vi "Strip Unit.vi"(8 "错误输入":errorcluster, 10 "Number or 1D array with units":variant) -> (0 "错误输出":errorcluster, 2 "Pure Number(s) (base units)":variant)   [LabVIEW 2012, in "TD Tools.lvlib"]
uses:
  TD Tools.lvlib
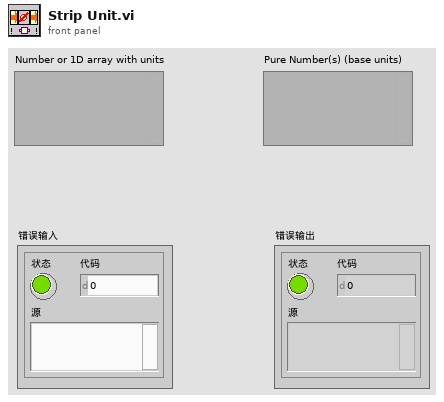
[diagram p1: front panel]
types:
  T1 = typedef "TD Tools.lvlib/Type Descriptor.ctl" = u16[]
  T2 = typedef "TD Tools.lvlib/Type Descriptor Header.ctl" = cluster{"length":u16, "private":u8, "type":T3, "# elements":u16}
  T3 = typedef "TD Tools.lvlib/Type Descriptor Enumeration.ctl" = enum16{"<Null>", "I8", "I16", "I32", "I64", "U8", "U16", "U32", "U64", "SGL", "DBL", "EXT", "CSG", "CDB", "CXT", "0x0F", "0x10", "0x11", "0x12", "0x13", "0x14", "Enum U8", "Enum U16", "Enum U32", "Enum U64", "SGL PQ", "DBL PQ", "EXT PQ", "CSG PQ", "CDB PQ", "CXT PQ", "0x1F", "0x20", "Boolean", "0x22", "0x23", "0x24", "0x25", "0x26", "0x27", "0x28", "0x29", "0x2A", "0x2B", "0x2C", "0x2D", "0x2E", "0x2F", "String", "0x31", "Path", "Pict", "0x34", "0x35", "0x36", "DAQ", "0x38", "0x39", "0x3A", "0x3B", "0x3C", "0x3D", "0x3E", "0x3F", "Array", "0x41", "0x42", "0x43", "0x44", "0x45", "0x46", "0x47", "0x48", "0x49", "0x4A", "0x4B", "0x4C", "0x4D", "0x4E", "0x4F", "Cluster", "0x51", "0x52", "Variant", "Waveform", "0x55", "0x56", "0x57", "0x58", "0x59", "0x5A", "0x5B", "0x5C", "0x5D", "0x5E", "0x5F", "0x60", "0x61", "0x62", "0x63", "0x64", "0x65", "0x66", "0x67", "0x68", "0x69", "0x6A", "0x6B", "0x6C", "0x6D", "0x6E", "0x6F", "Refnum"}
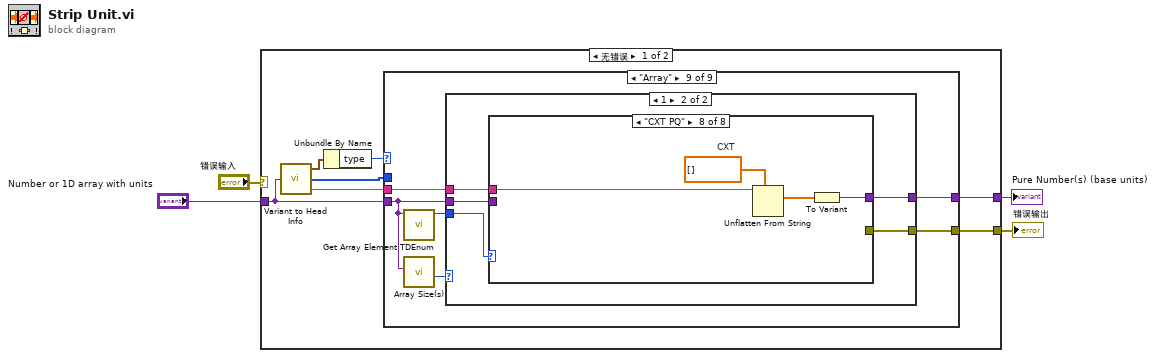
[diagram p0: block diagram]
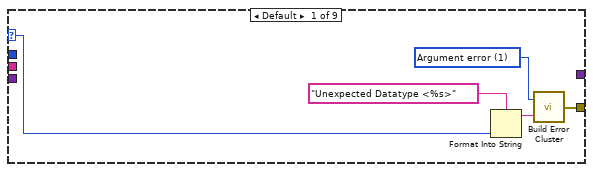
[diagram p2: hidden frame]
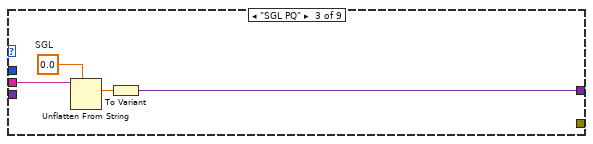
[diagram p4: hidden frame]
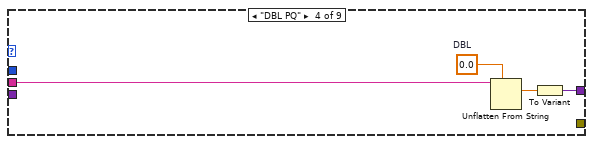
[diagram p5: hidden frame]
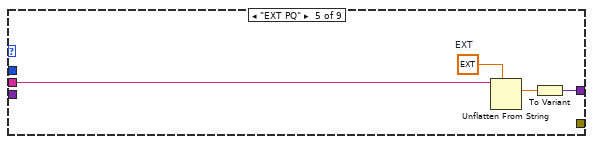
[diagram p6: hidden frame]
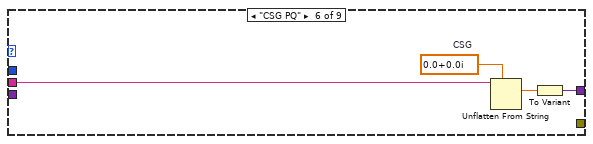
[diagram p7: hidden frame]
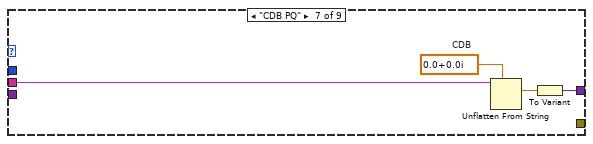
[diagram p8: hidden frame]
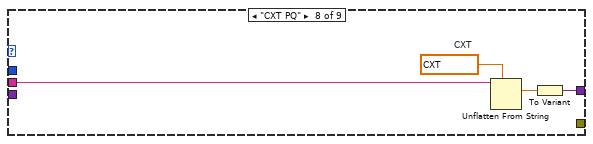
[diagram p9: hidden frame]
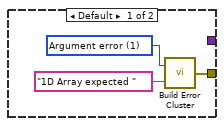
[diagram p10: hidden frame]
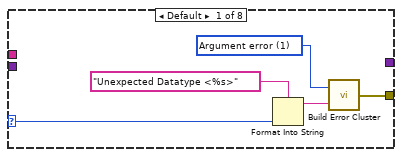
[diagram p11: hidden frame]
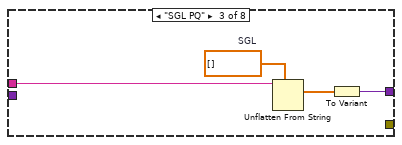
[diagram p13: hidden frame]
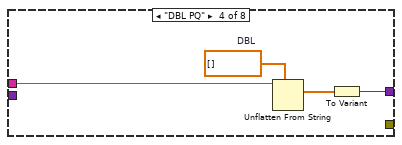
[diagram p14: hidden frame]
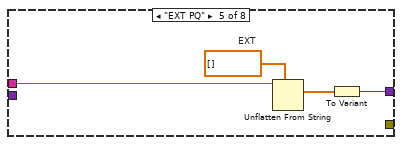
[diagram p15: hidden frame]
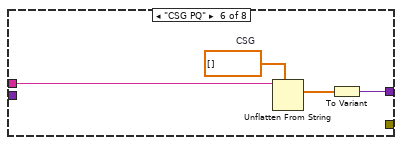
[diagram p16: hidden frame]
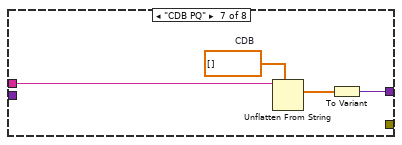
[diagram p17: hidden frame]
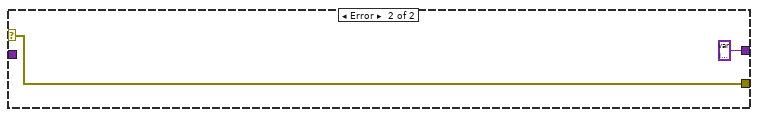
[diagram p18: hidden frame]
diagram:
  n1 = case shown="无错误" "错误输入" {
    selector: "错误输入" -> [_ w87]
    tunnel: [w11 w87] -> w2
    tunnel: "Number or 1D array with units" -> [w5 _]
    tunnel: [w6 variant ("Variant")] -> w3
    frame No Error {
      n2 = call "Variant to Head Info.vi"("Variant"=w5) -> ("Data String"=w7:string, "Type Descriptor"=w8:T1, "Type Descriptor Header"=w10:T2)  [unwired: 2 in]
      n3 = Unbundle By Name(w10) -> ("type"=w9:T3)
      n4 = case shown="\"Array\"" w9 {
        selector: w9 -> [w13 _ _ _ _ _ _ _ _]
        tunnel: [w16 _ _ _ _ _ _ _ w46] -> w11
        tunnel: w8 -> [_ _ _ _ _ _ _ _ _]
        tunnel: w7 -> [_ _ w18 w22 w26 w30 w34 w38 w44]
        tunnel: [_ w17 w19 w23 w27 w31 w35 w39 w45] -> w6
        tunnel: w5 -> [_ w17 _ _ _ _ _ _ w43]
        frame Default {
          w15 = 1 items=["No error", "Argument error", "Memory is full", "Out of zone", "End of file", "File already open", "Generic file I/O error", "File not found", "File permission error", "Disk is full", "Duplicate path", "Too many files open", "System feature not enabled", "Resource file not found", "Cannot add resource", "Resource not found", "Image not found", "Image memory error", "Pen does not exist", "Config type invalid", "Config token not found", "Config parse error", "Config memory error", "Bad external code format", "Bad external code offset", "External code not present", "Null window", "Destroy window error", "Null menu", "Print aborted", "Bad print record", "Print driver error", "Windows error during printing", "Memory error during printing", "Print dialog error", "Generic print error", "Invalid device refnum", "Device not found", "Device parameter error", "Device unit error", "Cannot open device", "Device call aborted", "Generic error", "Cancelled by user", "Object ID too low", "Object ID too high", "Object not in heap", "Unknown heap", "Unknown object (invalid DefProc)", "Unknown object (DefProc not in table)", "Message out of range", "Invalid (null) method", "Unknown message", "Manager call not supported", "Bad address", "Network operation in progress", "Network operation timed out", "Connection is busy", "Network attribute not supported", "Network error", "Address in use", "System out of memory", "Connection aborted", "Connection refused", "Not connected", "Already connected", "Connection closed", "Initialization error (interapplication manager)", "Bad occurrence", "Wait on unbound occurrence handler", "Occurrence queue overflow", "Datalog type conflict", "Unused", "Unrecognized type (interapplication manager)", "Memory corrupt", "Failed to make temporary DLL", "Old CIN version", "Drag socket not found", "Failed to load drop-object", "Failed to register OLE object", "Failed to release OLE object", "Format specifier type mismatch", "Unknown format specifier", "Too few format specifiers", "Too many format specifiers", "Scan failed", "Newer CIN version", "Error converting to variant", "Runtime menu error", "Password tampered", "Variant attribute not found", "Incompatible variant data type", "Event data is not available", "Event Store is not present", "Occurrence is not found", "Event Queue is not created", "Event info is not available", "Refnum passed is NULL", "Error retrieving Class GUID", "Error retrieving CoClass GUID", "Error retrieving TypeLib GUID.", "Bad built application magic bytes.", "Specific driver is different from the specific driver associated with the Logical Name.", "There is no session opened to the class driver.", "Max Error", "MAX - Error with config objects", "MAX - Error loading configuration", "MAX - Group not supported"]
          n5 = Format Into String(format string="Unexpected Datatype <%s>" ("Format String"), w13) -> (resulting string=w12:string)  [unwired: 2 in, 1 out]
          n6 = call "Build Error Cluster.vi"("String to Prepend to source (\"\")"=w12, "code"=w15) -> ("error out"=w16:errorcluster)
        }
        frame "SGL".."CXT" {
        }
        frame "SGL PQ" {
          w21 = sgl 0.0  # SGL
          n7 = Unflatten From String(type=w21, binary string=w18) -> (value=w20:sgl)  [unwired: 3 in, 2 out]
          n8 = To Variant(anything=w20) -> (Variant=w19:variant)
        }
        frame "DBL PQ" {
          w25 = 0.0  # DBL
          n9 = Unflatten From String(type=w25, binary string=w22) -> (value=w24:dbl)  [unwired: 3 in, 2 out]
          n10 = To Variant(anything=w24) -> (Variant=w23:variant)
        }
        frame "EXT PQ" {
          w29 = ext 0.0  # EXT
          n11 = Unflatten From String(type=w29, binary string=w26) -> (value=w28:ext)  [unwired: 3 in, 2 out]
          n12 = To Variant(anything=w28) -> (Variant=w27:variant)
        }
        frame "CSG PQ" {
          w33 = csg 0.0+0.0i  # CSG
          n13 = Unflatten From String(type=w33, binary string=w30) -> (value=w32:csg)  [unwired: 3 in, 2 out]
          n14 = To Variant(anything=w32) -> (Variant=w31:variant)
        }
        frame "CDB PQ" {
          w37 = cdb 0.0+0.0i  # CDB
          n15 = Unflatten From String(type=w37, binary string=w34) -> (value=w36:cdb)  [unwired: 3 in, 2 out]
          n16 = To Variant(anything=w36) -> (Variant=w35:variant)
        }
        frame "CXT PQ" {
          w41 = cxt 0.0+0.0i  # CXT
          n17 = Unflatten From String(type=w41, binary string=w38) -> (value=w40:cxt)  [unwired: 3 in, 2 out]
          n18 = To Variant(anything=w40) -> (Variant=w39:variant)
        }
        frame "Array" {
          n19 = call "Get Array Element TDEnum.vi"("Array"=w43) -> ("Type Code"=w47:T3)  [unwired: 9 in, 1 out]
          n20 = call "Array Size(s).vi"("Array"=w43) -> ("N dims"=w42:u32)  [unwired: 8 in, 2 out]
          n21 = case shown="1" w42 {
            tunnel: w47 -> [_ w55]
            tunnel: [w49 w54] -> w46
            tunnel: [_ w53] -> w45
            tunnel: w44 -> [_ w52]
            tunnel: w43 -> [_ w51]
            frame Default {
              w50 = 1 items=["No error", "Argument error", "Memory is full", "Out of zone", "End of file", "File already open", "Generic file I/O error", "File not found", "File permission error", "Disk is full", "Duplicate path", "Too many files open", "System feature not enabled", "Resource file not found", "Cannot add resource", "Resource not found", "Image not found", "Image memory error", "Pen does not exist", "Config type invalid", "Config token not found", "Config parse error", "Config memory error", "Bad external code format", "Bad external code offset", "External code not present", "Null window", "Destroy window error", "Null menu", "Print aborted", "Bad print record", "Print driver error", "Windows error during printing", "Memory error during printing", "Print dialog error", "Generic print error", "Invalid device refnum", "Device not found", "Device parameter error", "Device unit error", "Cannot open device", "Device call aborted", "Generic error", "Cancelled by user", "Object ID too low", "Object ID too high", "Object not in heap", "Unknown heap", "Unknown object (invalid DefProc)", "Unknown object (DefProc not in table)", "Message out of range", "Invalid (null) method", "Unknown message", "Manager call not supported", "Bad address", "Network operation in progress", "Network operation timed out", "Connection is busy", "Network attribute not supported", "Network error", "Address in use", "System out of memory", "Connection aborted", "Connection refused", "Not connected", "Already connected", "Connection closed", "Initialization error (interapplication manager)", "Bad occurrence", "Wait on unbound occurrence handler", "Occurrence queue overflow", "Datalog type conflict", "Unused", "Unrecognized type (interapplication manager)", "Memory corrupt", "Failed to make temporary DLL", "Old CIN version", "Drag socket not found", "Failed to load drop-object", "Failed to register OLE object", "Failed to release OLE object", "Format specifier type mismatch", "Unknown format specifier", "Too few format specifiers", "Too many format specifiers", "Scan failed", "Newer CIN version", "Error converting to variant", "Runtime menu error", "Password tampered", "Variant attribute not found", "Incompatible variant data type", "Event data is not available", "Event Store is not present", "Occurrence is not found", "Event Queue is not created", "Event info is not available", "Refnum passed is NULL", "Error retrieving Class GUID", "Error retrieving CoClass GUID", "Error retrieving TypeLib GUID.", "Bad built application magic bytes.", "Specific driver is different from the specific driver associated with the Logical Name.", "There is no session opened to the class driver.", "Max Error", "MAX - Error with config objects", "MAX - Error loading configuration", "MAX - Group not supported"]
              n22 = call "Build Error Cluster.vi"("String to Prepend to source (\"\")"="1D Array expected " ("Format String"), "code"=w50) -> ("error out"=w49:errorcluster)
            }
            frame 1 {
              n23 = case shown="\"CXT PQ\"" w55 {
                selector: w55 -> [w57 _ _ _ _ _ _ _]
                tunnel: [w56 _ _ _ _ _ _ _] -> w54
                tunnel: [_ w61 w62 w66 w70 w74 w78 w82] -> w53
                tunnel: w51 -> [_ w61 _ _ _ _ _ _]
                tunnel: w52 -> [_ _ w63 w67 w71 w75 w79 w83]
                frame Default {
                  w60 = 1 items=["No error", "Argument error", "Memory is full", "Out of zone", "End of file", "File already open", "Generic file I/O error", "File not found", "File permission error", "Disk is full", "Duplicate path", "Too many files open", "System feature not enabled", "Resource file not found", "Cannot add resource", "Resource not found", "Image not found", "Image memory error", "Pen does not exist", "Config type invalid", "Config token not found", "Config parse error", "Config memory error", "Bad external code format", "Bad external code offset", "External code not present", "Null window", "Destroy window error", "Null menu", "Print aborted", "Bad print record", "Print driver error", "Windows error during printing", "Memory error during printing", "Print dialog error", "Generic print error", "Invalid device refnum", "Device not found", "Device parameter error", "Device unit error", "Cannot open device", "Device call aborted", "Generic error", "Cancelled by user", "Object ID too low", "Object ID too high", "Object not in heap", "Unknown heap", "Unknown object (invalid DefProc)", "Unknown object (DefProc not in table)", "Message out of range", "Invalid (null) method", "Unknown message", "Manager call not supported", "Bad address", "Network operation in progress", "Network operation timed out", "Connection is busy", "Network attribute not supported", "Network error", "Address in use", "System out of memory", "Connection aborted", "Connection refused", "Not connected", "Already connected", "Connection closed", "Initialization error (interapplication manager)", "Bad occurrence", "Wait on unbound occurrence handler", "Occurrence queue overflow", "Datalog type conflict", "Unused", "Unrecognized type (interapplication manager)", "Memory corrupt", "Failed to make temporary DLL", "Old CIN version", "Drag socket not found", "Failed to load drop-object", "Failed to register OLE object", "Failed to release OLE object", "Format specifier type mismatch", "Unknown format specifier", "Too few format specifiers", "Too many format specifiers", "Scan failed", "Newer CIN version", "Error converting to variant", "Runtime menu error", "Password tampered", "Variant attribute not found", "Incompatible variant data type", "Event data is not available", "Event Store is not present", "Occurrence is not found", "Event Queue is not created", "Event info is not available", "Refnum passed is NULL", "Error retrieving Class GUID", "Error retrieving CoClass GUID", "Error retrieving TypeLib GUID.", "Bad built application magic bytes.", "Specific driver is different from the specific driver associated with the Logical Name.", "There is no session opened to the class driver.", "Max Error", "MAX - Error with config objects", "MAX - Error loading configuration", "MAX - Group not supported"]
                  n24 = Format Into String(format string="Unexpected Datatype <%s>" ("Format String"), w57) -> (resulting string=w58:string)  [unwired: 2 in, 1 out]
                  n25 = call "Build Error Cluster.vi"("String to Prepend to source (\"\")"=w58, "code"=w60) -> ("error out"=w56:errorcluster)
                }
                frame "SGL".."CXT" {
                }
                frame "SGL PQ" {
                  w64 = sgl[] []  # SGL
                  n26 = Unflatten From String(type=w64, binary string=w63) -> (value=w65:sgl[])  [unwired: 3 in, 2 out]
                  n27 = To Variant(anything=w65) -> (Variant=w62:variant)
                }
                frame "DBL PQ" {
                  w68 = dbl[] []  # DBL
                  n28 = Unflatten From String(type=w68, binary string=w67) -> (value=w69:dbl[])  [unwired: 3 in, 2 out]
                  n29 = To Variant(anything=w69) -> (Variant=w66:variant)
                }
                frame "EXT PQ" {
                  w72 = ext[] []  # EXT
                  n30 = Unflatten From String(type=w72, binary string=w71) -> (value=w73:ext[])  [unwired: 3 in, 2 out]
                  n31 = To Variant(anything=w73) -> (Variant=w70:variant)
                }
                frame "CSG PQ" {
                  w76 = csg[] []  # CSG
                  n32 = Unflatten From String(type=w76, binary string=w75) -> (value=w77:csg[])  [unwired: 3 in, 2 out]
                  n33 = To Variant(anything=w77) -> (Variant=w74:variant)
                }
                frame "CDB PQ" {
                  w80 = cdb[] []  # CDB
                  n34 = Unflatten From String(type=w80, binary string=w79) -> (value=w81:cdb[])  [unwired: 3 in, 2 out]
                  n35 = To Variant(anything=w81) -> (Variant=w78:variant)
                }
                frame "CXT PQ" {
                  w84 = cxt[] []  # CXT
                  n36 = Unflatten From String(type=w84, binary string=w83) -> (value=w85:cxt[])  [unwired: 3 in, 2 out]
                  n37 = To Variant(anything=w85) -> (Variant=w82:variant)
                }
              }
            }
          }
        }
      }
    }
    frame Error {
    }
  }
  "Pure Number(s) (base units)" <- w3
  "错误输出" <- w2
